vi "Bit Manipulation.vi"(5 "Field Value (0)":i32, 6 "Width (1)":i32=1, 7 "Bit Index (1)":i32=1, 8 "error in (no error)":errorcluster, 9 "Number (0)":i32, 10 "Operation (0: Clear Bit)":i32(ring) items=["Clear Bit", "Get Bit", "Get Field Bits", "Set Bit", "Set Field Bits", "Test Bit", "Toggle Bit"], 11 "VISA resource name":refnum<visa-resource-name>) -> (0 "error out":errorcluster, 2 "Result":i32, 3 "VISA resource name out":refnum<visa-resource-name>)   [LabVIEW 2020, in "Keithley 2600 Series.lvlib"]
doc: "Performs a bitwise calculation on one number."
uses:
  <instrlib>/Keithley 2600 Series/Keithley 2600 Series.lvlib
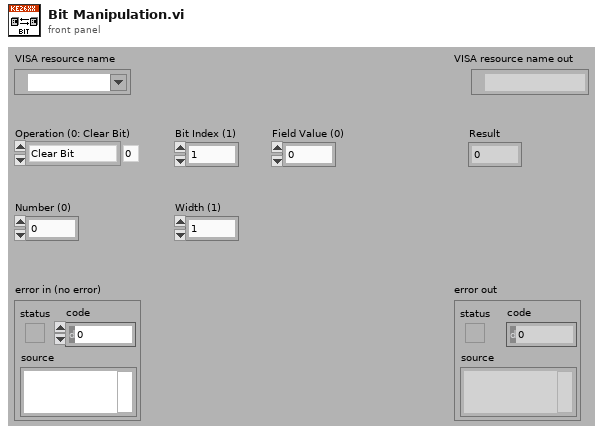
[diagram p1: front panel]
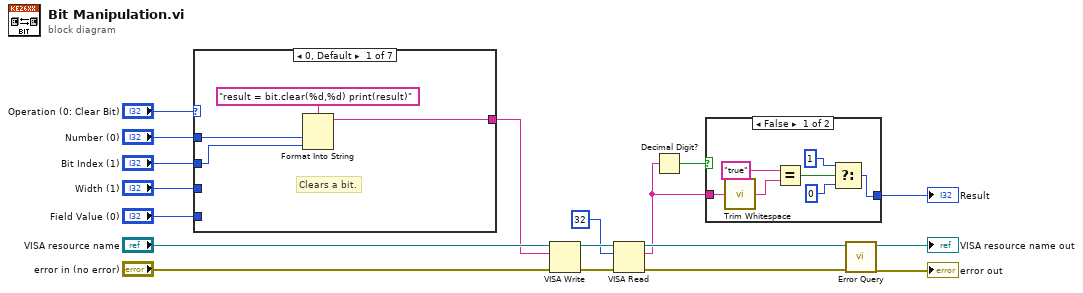
[diagram p0: block diagram]
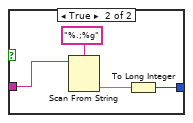
[diagram p2: hidden frame]
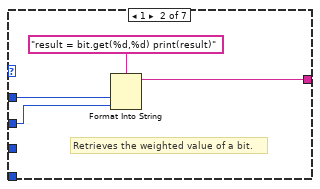
[diagram p3: hidden frame]
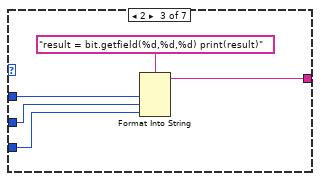
[diagram p4: hidden frame]
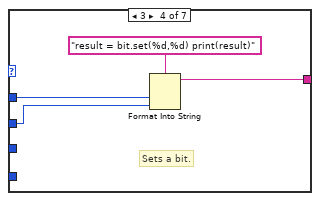
[diagram p5: hidden frame]
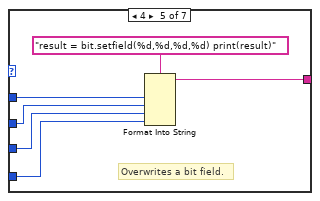
[diagram p6: hidden frame]
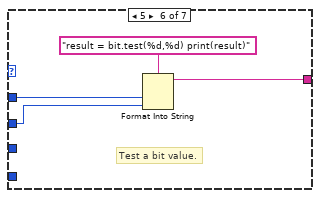
[diagram p7: hidden frame]
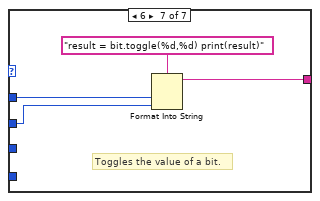
[diagram p8: hidden frame]
diagram:
  n1 = case shown="0, Default" "Operation (0: Clear Bit)" {
    tunnel: "Number (0)" -> [w21 w25 w30 w34 w40 w44 w48]
    tunnel: "Bit Index (1)" -> [w20 w24 w29 w33 w39 w43 w47]
    tunnel: "Width (1)" -> [_ _ w27 _ w36 _ _]
    tunnel: "Field Value (0)" -> [_ _ _ _ w37 _ _]
    tunnel: [w19 w23 w28 w32 w38 w42 w46] -> w4
    frame 0, Default {
      # "Clears a bit."
      n2 = Format Into String(format string="result = bit.clear(%d,%d) print(result)", w21, w20) -> (resulting string=w19:string)  [unwired: 2 in, 1 out]
    }
    frame 1 {
      # "Retrieves the weighted value of a bit."
      n3 = Format Into String(format string="result = bit.get(%d,%d) print(result)", w25, w24) -> (resulting string=w23:string)  [unwired: 2 in, 1 out]
    }
    frame 2 {
      n4 = Format Into String(format string="result = bit.getfield(%d,%d,%d) print(result)", w30, w29, w27) -> (resulting string=w28:string)  [unwired: 2 in, 1 out]
    }
    frame 3 {
      # "Sets a bit."
      n5 = Format Into String(format string="result = bit.set(%d,%d) print(result)", w34, w33) -> (resulting string=w32:string)  [unwired: 2 in, 1 out]
    }
    frame 4 {
      # "Overwrites a bit field."
      n6 = Format Into String(format string="result = bit.setfield(%d,%d,%d,%d) print(result)", w40, w39, w36, w37) -> (resulting string=w38:string)  [unwired: 2 in, 1 out]
    }
    frame 5 {
      # "Test a bit value."
      n7 = Format Into String(format string="result = bit.test(%d,%d) print(result)", w44, w43) -> (resulting string=w42:string)  [unwired: 2 in, 1 out]
    }
    frame 6 {
      # "Toggles the value of a bit."
      n8 = Format Into String(format string="result = bit.toggle(%d,%d) print(result)", w48, w47) -> (resulting string=w46:string)  [unwired: 2 in, 1 out]
    }
  }
  n9 = VISA Write(VISA resource name="VISA resource name", write buffer=w4, error in (no error)="error in (no error)") -> (VISA resource name out=w14:refnum<visa-resource-name>, error out=w12:errorcluster)  [unwired: 1 out]
  n10 = VISA Read(VISA resource name=w14, byte count=u32 32, error in (no error)=w12) -> (VISA resource name out=w13:refnum<visa-resource-name>, read buffer=w2:string, error out=w11:errorcluster)  [unwired: 1 out]
  n11 = Decimal Digit?(1:w2) -> (0:w3:bool)
  n12 = case shown="False" w3 {
    tunnel: w2 -> [w51 w59]
    tunnel: [w56 w58] -> w1
    frame False {
      n13 = call <vilib>:"Trim Whitespace.vi"("string"=w51) -> ("trimmed string"=w50:string)  [unwired: 1 in]
      n14 = Equal?(x="true", y=w50) -> (x = y?=w55:bool)
      n15 = Select(t=1, s=w55, f=0) -> (s? t:f=w56:i32)
    }
    frame True {
      n16 = Scan From String(format string="%.;%g", input string=w59) -> (output 1=w57:dbl)  [unwired: 3 in, 3 out]
      n17 = To Long Integer(number=w57) -> (32bit integer=w58:i32)
    }
  }
  "Result" <- w1
  n18 = call <instrlib>:"Error Query.vi"("error in (no error)"=w11, "VISA resource name"=w13) -> ("error out"=→"error out":errorcluster, "VISA resource name out"=→"VISA resource name out":refnum<visa-resource-name>)  [unwired: 6 in, 2 out]
